vi "Raycaster_DrawColumnSimple.vi"(4 "Sub Buffer":u8, 6 "column":u32, 8 "Buffer In":u8[](array[numeric]), 10 "Column Calcs":T1, 11 "DDA Calculation In":T2) -> (0 "Buffer Out":u8[](array[numeric]))   [LabVIEW 2020]
uses:
  Controls/Raycaster_DDACalcs.ctl
  Controls/Raycaster_WallColumnAxis.ctl
  Controls/Raycaster_ScreenCalcs.ctl
  <vilib>/rvi/DataTransferAndStorage/Container/XNode/niFpgaContainer.xnode
  <vilib>/rvi/DataTransferAndStorage/Register/Emulation/niFpgaRegisterEmulation.vi
  <vilib>/Platform/TimedLoop/XDataNode/XDataNode.xnode
  <vilib>/Platform/TimedLoop/XDataNode/nitl_modes.ctl
  <vilib>/Platform/TimedLoop/XDataNode/XDNodeRunTimeDep.lvlib
  <vilib>/Platform/TimedLoop/XDataNode/wakeup.ctl
  <vilib>/Platform/TimedLoop/XDataNode/timing_clust.ctl
  <vilib>/rvi/Memory/Memory_Emulation/nirvimemoryFastEmulation.vi
  <vilib>/rvi/Memory/Memory_Emulation/nirvimemoryEmulation.vi
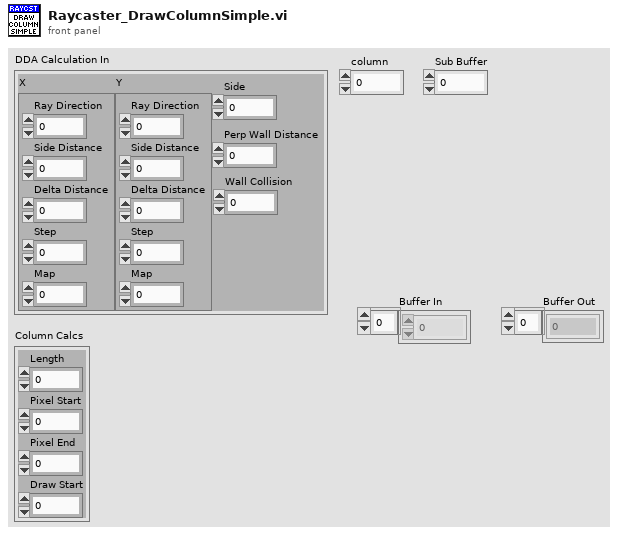
[diagram p1: front panel]
types:
  T1 = typedef "Raycaster_ScreenCalcs.ctl" = cluster{"Length":i16, "Pixel Start":i16, "Pixel End":i16, "Draw Start":i16}
  T2 = typedef "Raycaster_DDACalcs.ctl" = cluster{"X":T3, "Y":T3, "Side":u8, "Perp Wall Distance":fxp<+/-,32,16>, "Wall Collision":u8}
  T3 = typedef "Raycaster_WallColumnAxis.ctl" = cluster{"Ray Direction":fxp<+/-,32,16>, "Side Distance":fxp<+/-,32,16>, "Delta Distance":fxp<+/-,32,16>, "Step":i16, "Map":i16}
  T4 = typedef "XDNodeRunTimeDep.lvlib/timing_clust.ctl" = cluster{"Expected End [f-1]":u64, "Actual End [f-1]":u64, "Finished Late? [f-1]":bool, "Expected End [i-1]":u64, "Actual End [i-1]":u64, "Finished Late? [i-1]":bool, "Expected Start [i]":u64, "Actual Start [i]":u64, "Expected Start [f]":u64, "Actual Start [f]":u64, "Source Name":string, "Structure Name":string, "Period":i64, "Deadline":i64, "Offset":i64, "Start":i64, "Priority":i32, "Timeout":i32, "Mode":T5, "Wakeup Reason":T6, "Error":errorcluster, "Source Type":string, "Secondary Source Type":string, "Global End Time":u64, "Global Start Time":u64, "Frame Duration":u64, "Iteration Duration":u64, "Assigned CPU":i32, "I/O Scan Engine Mode":u32}
  T5 = typedef "XDNodeRunTimeDep.lvlib/nitl_modes.ctl" = enum32{"No Change", "Process missed periods, maintain original phase", "Discard missed periods, maintain original phase", "Process missed periods, ignore original phase", "Discard missed periods, ignore original phase"}
  T6 = typedef "XDNodeRunTimeDep.lvlib/wakeup.ctl" = enum32{"Normal", "Aborted", "Asynchronous wakeup", "Timing source error", "Timed loop error", "Timeout"}
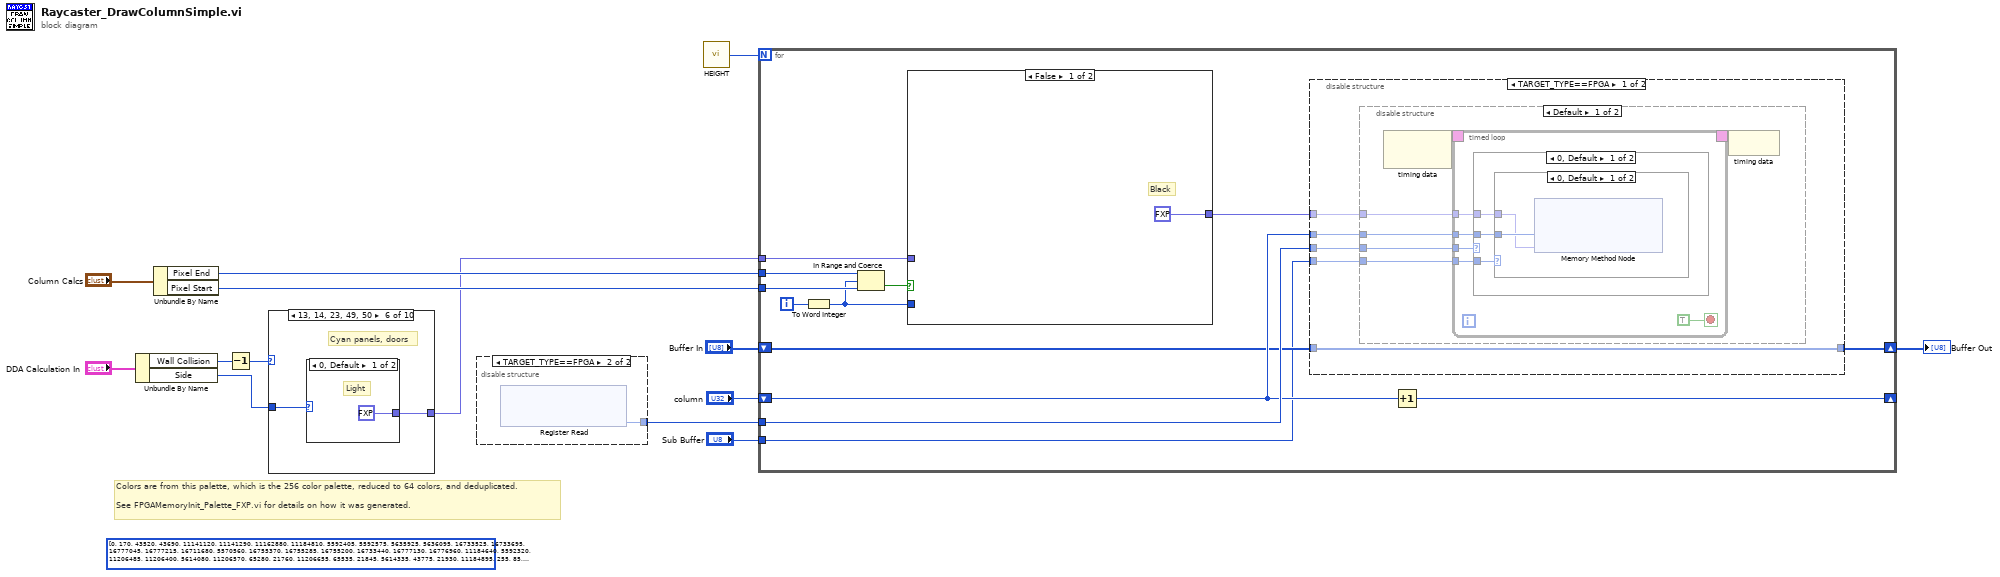
[diagram p0: block diagram]
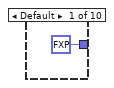
[diagram p2: hidden frame]
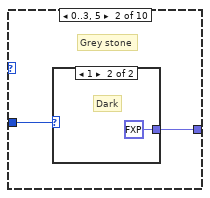
[diagram p3: hidden frame]
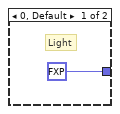
[diagram p4: hidden frame]
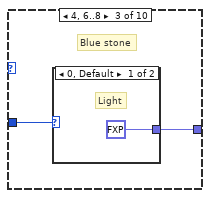
[diagram p5: hidden frame]
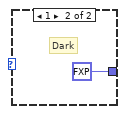
[diagram p6: hidden frame]
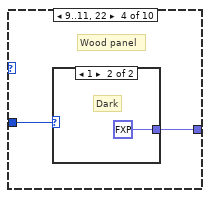
[diagram p7: hidden frame]
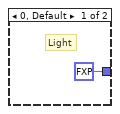
[diagram p8: hidden frame]
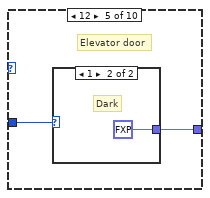
[diagram p9: hidden frame]
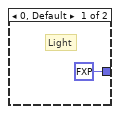
[diagram p10: hidden frame]
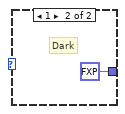
[diagram p11: hidden frame]
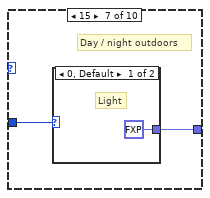
[diagram p12: hidden frame]
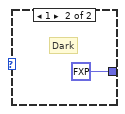
[diagram p13: hidden frame]
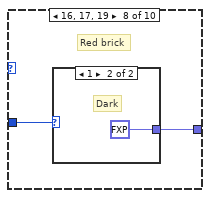
[diagram p14: hidden frame]
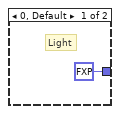
[diagram p15: hidden frame]
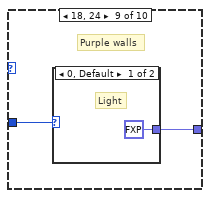
[diagram p16: hidden frame]
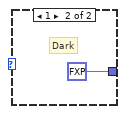
[diagram p17: hidden frame]
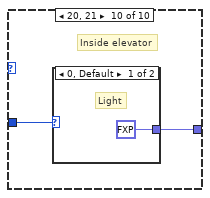
[diagram p18: hidden frame]
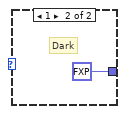
[diagram p19: hidden frame]
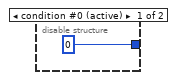
[diagram p20: hidden frame]
diagram:
  (unwired) u32[] [0, 170, 43520, 43690, 11141120, 11141290, 11162880, 11184810, 5592405, 5592575, 5635925, 5636095, 16733525, 16733695, 16777045, 16777215, 16711680, 5570560, 16755370, 16755285, 16755200, 16733440, 16777130, 16776960, 11184640, 5592320, 11206485, 11206400, 5614080, 11206570, 65280, 21760, 11206655, 65535, 21845, 5614335, 43775, 21930, 11184895, 255, 85, 11141375, 5570730, 5570645, 16755455, 16711935, 11184725, 11162965, 5614250] ("Palette")
  # "Colors are from this palette, which is the 256 color palette, reduced to 64 colors, and deduplicated.\n\nSee FPGAMemoryInit_Palette_FXP.vi for details on how it was generated."
  n1 = Unbundle By Name("DDA Calculation In") -> ("Wall Collision"=w4:u8, "Side"=w3:u8)
  n2 = Unbundle By Name("Column Calcs") -> ("Pixel End"=w6:i16, "Pixel Start"=w5:i16)
  n3 = Decrement(x=w4) -> (x-1=w1:u8)
  n4 = case shown="13, 14, 23, 49, 50" w1 {
    tunnel: w3 -> [_ w17 w21 w25 w29 w33 w37 w41 w45 w49]
    tunnel: [fxp<+,6,6> 14.0 w16 w20 w24 w28 w32 w36 w40 w44 w48] -> w2
    frame Default {
    }
    frame 0..3, 5 {
      # "Grey stone"
      n5 = case shown="1" w17 {
        tunnel: [fxp<+,6,6> 7.0 fxp<+,6,6> 8.0] -> w16
        frame 0, Default {
          # "Light"
        }
        frame 1 {
          # "Dark"
        }
      }
    }
    frame 4, 6..8 {
      # "Blue stone"
      n6 = case shown="0, Default" w21 {
        tunnel: [fxp<+,6,6> 39.0 fxp<+,6,6> 1.0] -> w20
        frame 0, Default {
          # "Light"
        }
        frame 1 {
          # "Dark"
        }
      }
    }
    frame 9..11, 22 {
      # "Wood panel"
      n7 = case shown="1" w25 {
        tunnel: [fxp<+,6,6> 6.0 fxp<+,6,6> 17.0] -> w24
        frame 0, Default {
          # "Light"
        }
        frame 1 {
          # "Dark"
        }
      }
    }
    frame 12 {
      # "Elevator door"
      n8 = case shown="1" w29 {
        tunnel: [fxp<+,6,6> 7.0 fxp<+,6,6> 8.0] -> w28
        frame 0, Default {
          # "Light"
        }
        frame 1 {
          # "Dark"
        }
      }
    }
    frame 13, 14, 23, 49, 50 {
      # "Cyan panels, doors"
      n9 = case shown="0, Default" w33 {
        tunnel: [fxp<+,6,6> 33.0 fxp<+,6,6> 3.0] -> w32
        frame 0, Default {
          # "Light"
        }
        frame 1 {
          # "Dark"
        }
      }
    }
    frame 15 {
      # "Day / night outdoors"
      n10 = case shown="0, Default" w37 {
        tunnel: [fxp<+,6,6> 0.0 fxp<+,6,6> 0.0] -> w36
        frame 0, Default {
          # "Light"
        }
        frame 1 {
          # "Dark"
        }
      }
    }
    frame 16, 17, 19 {
      # "Red brick"
      n11 = case shown="1" w41 {
        tunnel: [fxp<+,6,6> 16.0 fxp<+,6,6> 4.0] -> w40
        frame 0, Default {
          # "Light"
        }
        frame 1 {
          # "Dark"
        }
      }
    }
    frame 18, 24 {
      # "Purple walls"
      n12 = case shown="0, Default" w45 {
        tunnel: [fxp<+,6,6> 5.0 fxp<+,6,6> 42.0] -> w44
        frame 0, Default {
          # "Light"
        }
        frame 1 {
          # "Dark"
        }
      }
    }
    frame 20, 21 {
      # "Inside elevator"
      n13 = case shown="0, Default" w49 {
        tunnel: [fxp<+,6,6> 8.0 fxp<+,6,6> 7.0] -> w48
        frame 0, Default {
          # "Light"
        }
        frame 1 {
          # "Dark"
        }
      }
    }
  }
  n14 = disable-structure shown="TARGET_TYPE==FPGA" {
    disable-tunnel: [u8 0 ("Data") w53] -> w10
    frame condition #0 (active) {
    }
    frame condition #1 {
      n15 = xnode ("Register Read")() -> ("Data"=w53:u8)  [unwired: 1 in, 1 out]
    }
  }
  n16 = call "HEIGHT.vi"() -> ("HEIGHT"=w12:i16)
  n17 = for {
    N: w12 -> [_]
    tunnel: w5 -> [w65]
    tunnel: w6 -> [w64]
    tunnel: w10 -> [w60]
    shift-right: [w62] -> _
    shift-left: "column" -> [w59]
    tunnel: w2 -> [w61]
    shift-right: [w56] -> w8
    shift-left: "Buffer In" -> [w57]
    tunnel: "Sub Buffer" -> [w55]
    i -> [w66]
    n18 = To Word Integer(number=w66) -> (16bit integer=w54:i16)
    n19 = In Range and Coerce(upper limit=w64, x=w54, lower limit=w65) -> (In Range?=w63:bool)  [unwired: 1 out]
    n20 = case shown="False" w63 {
      tunnel: [fxp<+,6,6> 0.0 w68] -> w58
      tunnel: w61 -> [_ w68]
      tunnel: w54 -> [_ _]
      frame False {
        # "Black"
      }
      frame True {
      }
    }
    n21 = disable-structure shown="TARGET_TYPE==FPGA" {
      disable-tunnel: w59 -> [w71 w123]
      disable-tunnel: w57 -> [w73 w125]
      disable-tunnel: [w73 w124] -> w56
      disable-tunnel: w60 -> [w72 _]
      disable-tunnel: w58 -> [w70 w122]
      disable-tunnel: w55 -> [w69 _]
      frame condition #0 {
        n22 = disable-structure shown="Default" {
          disable-tunnel: w72 -> [w77 w106]
          disable-tunnel: w71 -> [w76 w105]
          disable-tunnel: w70 -> [w75 w104]
          disable-tunnel: w69 -> [w74 w103]
          frame condition #0 (active) {
            n23 = node-c288() -> (w79:T4)  [unwired: 1 in]
            n24 = timed-loop {
              timing: w79 -> [_]
              timing-out: [_] -> w78
              tunnel: w77 -> [w83]
              tunnel: w76 -> [w82]
              tunnel: w75 -> [w81]
              tunnel: w74 -> [w80]
              stop <- TRUE stop-if-true
              n25 = case shown="0, Default" w83 {
                tunnel: w82 -> [w87 w94]
                tunnel: w81 -> [w86 w93]
                tunnel: w80 -> [w85 w92]
                frame 0, Default {
                  n26 = case shown="0, Default" w85 {
                    tunnel: w87 -> [w89 w91]
                    tunnel: w86 -> [w88 w90]
                    frame 0, Default {
                      n27 = xnode ("Memory Method Node")("Address"=w89, "Data"=w88) -> ()  [unwired: 1 in, 1 out]
                    }
                    frame 1 {
                      n28 = xnode ("Memory Method Node")("Address"=w91, "Data"=w90) -> ()  [unwired: 1 in, 1 out]
                    }
                  }
                }
                frame 1 {
                  n29 = case shown="0, Default" w92 {
                    tunnel: w94 -> [w96 w98]
                    tunnel: w93 -> [w95 w97]
                    frame 0, Default {
                      n30 = xnode ("Memory Method Node")("Address"=w96, "Data"=w95) -> ()  [unwired: 1 in, 1 out]
                    }
                    frame 1 {
                      n31 = xnode ("Memory Method Node")("Address"=w98, "Data"=w97) -> ()  [unwired: 1 in, 1 out]
                    }
                  }
                }
              }
            }
            n32 = node-c288(w78) -> ()
          }
          frame condition #1 {
            n33 = node-c288() -> (w108:T4)  [unwired: 1 in]
            n34 = timed-loop {
              timing: w108 -> [_]
              timing-out: [_] -> w107
              tunnel: w106 -> [w112]
              tunnel: w105 -> [w111]
              tunnel: w104 -> [w110]
              tunnel: w103 -> [w109]
              stop <- TRUE stop-if-true
              n35 = case shown="0, Default" w112 {
                tunnel: w111 -> [w115 w117]
                tunnel: w110 -> [w114 w116]
                tunnel: w109 -> [_ _]
                frame 0, Default {
                  n36 = xnode ("Memory Method Node")("Address"=w115, "Data"=w114) -> ()  [unwired: 1 in, 1 out]
                }
                frame 1 {
                  n37 = xnode ("Memory Method Node")("Address"=w117, "Data"=w116) -> ()  [unwired: 1 in, 1 out]
                }
              }
            }
            n38 = node-c288(w107) -> ()
          }
        }
      }
      frame condition #1 (active) {
        n39 = Replace Array Subset(array=w125, new element=w122, index=w123) -> (w124:u8[])
      }
    }
    n40 = Increment(x=w59) -> (x+1=w62:u32)
  }
  "Buffer Out" <- w8
